vi "Kill RP proccess.vi"(8 "Error In":errorcluster) -> (0 "Error Out":errorcluster)   [LabVIEW 2016]
panel:
  in  "Password":string="changeme"
  out "Server  output":string
  in  "Process name":string="trd_rp"
  in  "Current address":string="192.168.1.100"
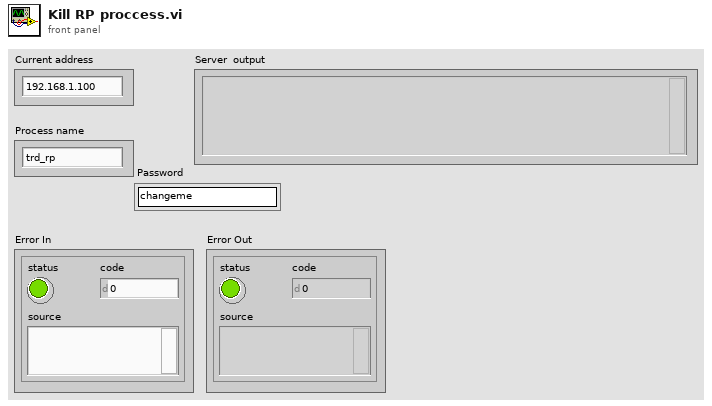
[diagram p1: front panel]
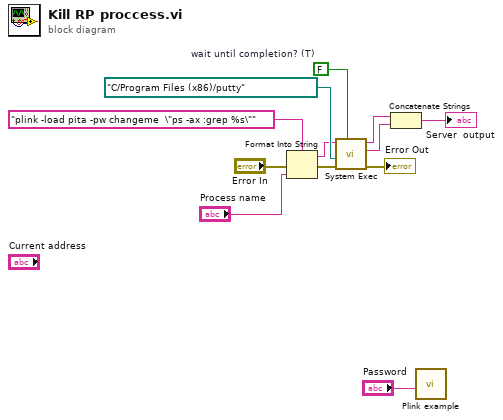
[diagram p0: block diagram]
diagram:
  w2 = FALSE  # wait until completion? (T)
  n1 = Format Into String(format string="plink -load pita -pw changeme  \"ps -ax :grep %s\"" ("command line"), error in="Error In", "Process name") -> (resulting string=w5:string, error out=w6:errorcluster)  [unwired: 1 in]
  n2 = call <vilib>:"System Exec.vi"("wait until completion? (T)"=w2, "error in (no error)"=w6, "working directory"=path "C:/Program Files (x86)/putty", "command line"=w5) -> ("error out"=→"Error Out":errorcluster, "standard error"=w9:string, "standard output"=w12:string)  [unwired: 4 in, 1 out]
  n3 = Concatenate Strings(w12, w9) -> (→"Server  output":string)
  n4 = call "Plink example.vi"("Password"="Password") -> ()  [unwired: 10 in, 1 out]
